vi "Load_Analogue_Data_2_Time_traces.vi"(0 "Sampling Rate (Hz)":dbl[](array[numeric]), 1 "Mode":T1, 2 "Index":i32[](array[numeric]), 3 "Voltage Array":dbl[][](array[numeric]), 4 "Time Trace":T2[](array[typedef]), 5 "Metadata Names":string[][](array[string]), 6 "Metadata Values":string[][](array[string])) -> ()   [LabVIEW 2021]
uses:
  Controls/Time_Trace_Cluster.ctl
  Sub_vis/Upload Data.ctl
  Globals/Meas_global.vi
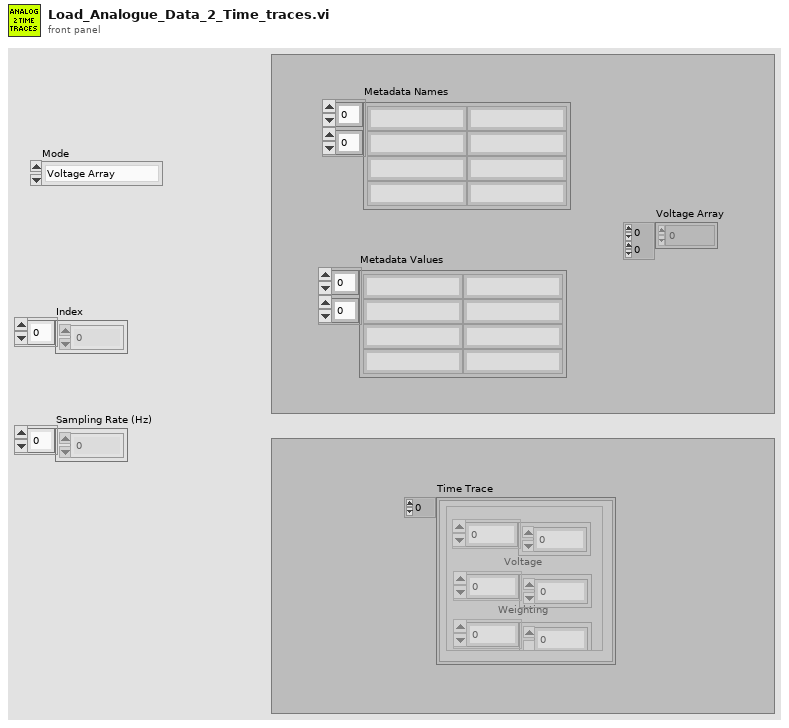
[diagram p1: front panel]
types:
  T1 = typedef "Upload Data.ctl" = enum16{"Voltage Array", "Time Trace Cluster"}
  T2 = typedef "Time_Trace_Cluster.ctl" = cluster{"Weighting":dbl[], "Voltage":dbl[], "Eng Values":dbl[]}
  T3 = typedef "Analysis_info_cluster.ctl" = cluster{"Colour":u32, "Inst type":T4, "Inst name":string, "Symbol":string, "Code name":string, "Extra Info":string, "Inst Array":T5, "Extra Titles":string[], "Extra Values":string[], "U":dbl, "u^2":dbl, "u^3":dbl, "u^4":dbl, "Skew_u":dbl, "Kurt_u":dbl, "Sd Error in Mean":dbl, "% u'/U":dbl, "X":dbl, "Y":dbl, "Z":dbl, "Timescale integral Estimate":dbl, "Sd Error in Variance":dbl, "Calib File":path, "Calib Constants":dbl[], "Output Position":bool, "Stats":enum16{"None", "Basic", "Full"}, "Av Sampling Rate":dbl, "Av No of Samples":dbl, "Total Meas Time (s)":dbl, "ADAM Ch Name":string, "Max value":dbl, "Min value":dbl, "Req Sample Rate Hz":dbl, "Sync Delay Time (s)":dbl, "Ch No":i16, "Device":string, "Use Latest Calib":bool, "Port":string, "Metadata Ch Names":string[], "Metadata Ch Values":string[], "Label":string}
  T4 = typedef "Inst_type.ctl" = enum16{"Raw voltage", "Raw with zero offsetting", "Propeller anemometer", "Pressure Transducer", "Pitot-static tube", "Hot wire", "Cross wire 1", "Cross wire 2", "Generic Linear", "Generic Polynomial", "Generic BackPoly", "Fast FID", "Thermocouple", "Cold wire", "Pulsed Wire", "LDA Vel", "LDA Tran time", "LDA Arr time", "Microphone"}
  T5 = typedef "Instrument_Array.ctl" = enum16{"PWA", "LDA", "Analogue"}
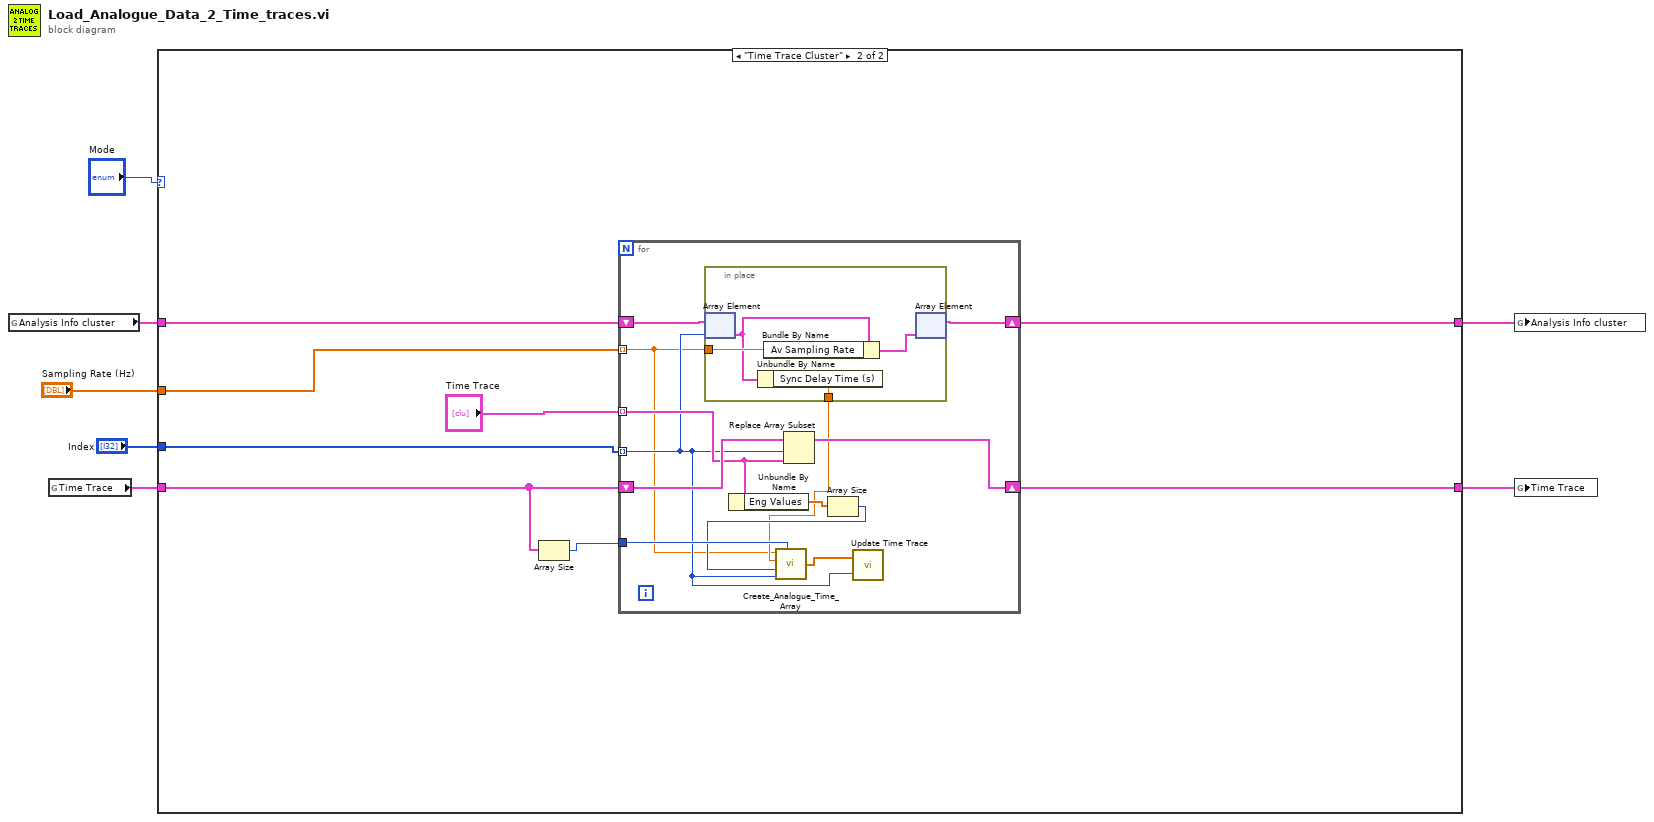
[diagram p0: block diagram]
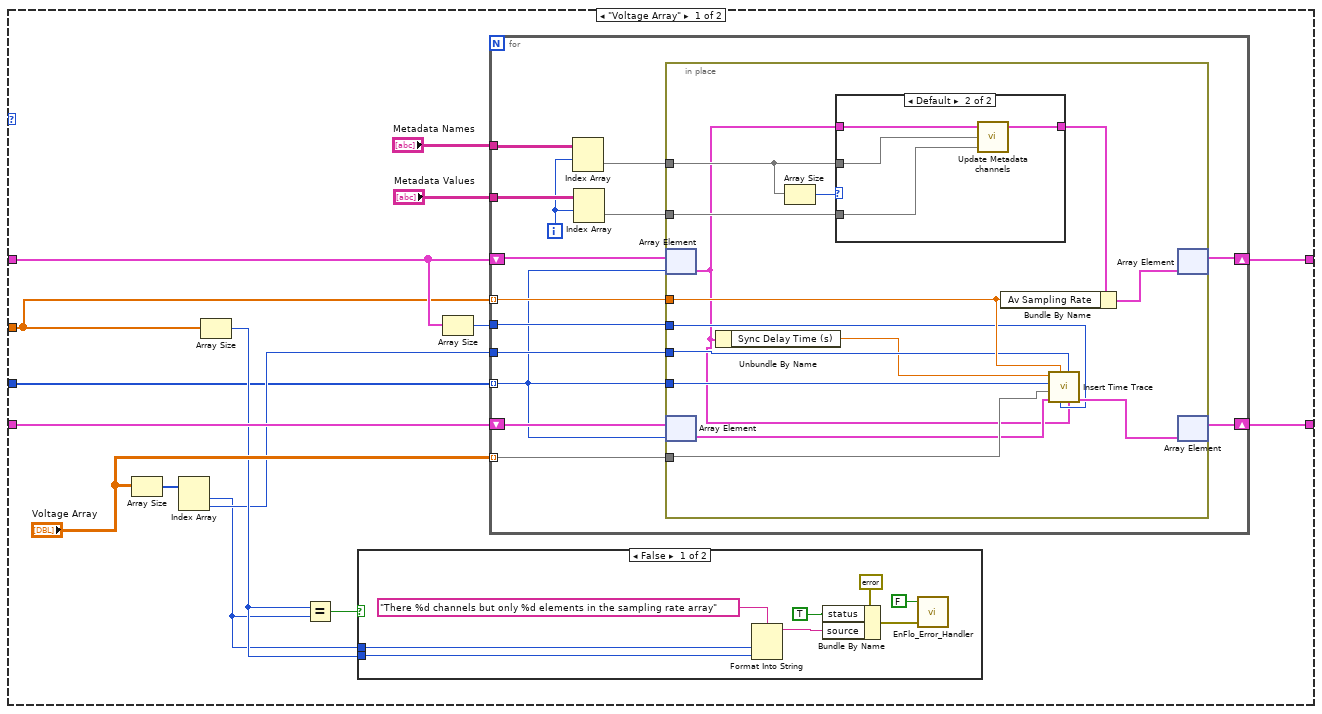
[diagram p2: hidden frame]
diagram:
  n1 = global read "Meas_global.vi" "Analysis Info cluster"() -> (w4:T3[])
  n2 = global read "Meas_global.vi" "Time Trace"() -> (w6:T2[])
  n3 = case shown="\"Time Trace Cluster\"" "Mode" {
    tunnel: [w22 w69] -> w7
    tunnel: w6 -> [w21 w65]
    tunnel: [w14 w70] -> w5
    tunnel: w4 -> [w13 w71]
    tunnel: "Sampling Rate (Hz)" -> [w9 w68]
    tunnel: "Index" -> [w8 w66]
    frame "Voltage Array" {
      n4 = Array Size(array="Voltage Array") -> (size(s)=w19:i32[])
      n5 = Index Array(array=w19) -> (element #1=w15:i32, element #2=w16:i32)  [unwired: 2 in]
      n6 = Array Size(array=w9) -> (size(s)=w17:i32)
      n7 = Equal?(x=w17, y=w15) -> (x = y?=w18:bool)
      n8 = case shown="False" w18 {
        tunnel: w15 -> [w27 _]
        tunnel: w17 -> [w26 _]
        frame False {
          n9 = Format Into String(format string="There %d channels but only %d elements in the sampling rate array", w27, w26) -> (resulting string=w24:string)  [unwired: 2 in, 1 out]
          n10 = Bundle By Name(cluster=errorcluster {"status"=FALSE, "code"=0, "source"=""} ("error in (no error)"), "status"=TRUE, "source"=w24) -> (w23:errorcluster)
          n11 = call "EnFlo_Error_Handler.vi"("error in (no error)"=w23, "Dialog Box (F)"=FALSE ("Dialog Box (T)")) -> ()  [unwired: 2 in, 2 out]
        }
        frame True {
        }
      }
      n12 = Array Size(array=w13) -> (size(s)=w12:i32)
      n13 = for {
        shift-right: [w42] -> w22
        shift-left: w21 -> [w44]
        tunnel: w8 -> [w36] mode=indexing
        tunnel: "Voltage Array" -> [w43] mode=indexing
        tunnel: w9 -> [w41] mode=indexing
        tunnel: w16 -> [w40]
        tunnel: w12 -> [w39]
        shift-right: [w37] -> w14
        shift-left: w13 -> [w38]
        tunnel: "Metadata Names" -> [w32]
        tunnel: "Metadata Values" -> [w35]
        i -> [w33]
        n14 = Index Array(array=w32, index (row)=w33) -> (element=w31:string[])  [unwired: 1 in]
        n15 = Index Array(array=w35, index (row)=w33) -> (element=w34:string[])  [unwired: 1 in]
        n16 = in-place {
          in-place-border: w43 -> [w53]
          in-place-border: w41 -> [w50]
          in-place-border: w40 -> [w49]
          in-place-border: w39 -> [w46]
          in-place-border: w36 -> [w47]
          in-place-border: w31 -> [w55]
          in-place-border: w34 -> [w57]
          n17 = in-place-array #1(w38, w36) -> (w45:T3)
          n18 = in-place-array #2(w44, w36) -> (w52:T2)
          n19 = Unbundle By Name(w45) -> ("Sync Delay Time (s)"=w48:dbl)
          n20 = Array Size(array=w55) -> (size(s)=w54:i32)
          n21 = case shown="Default" w54 {
            tunnel: w45 -> [w59 w63]
            tunnel: w57 -> [_ w60]
            tunnel: [w59 w62] -> w56
            tunnel: w55 -> [_ w61]
            frame 0 {
            }
            frame Default {
              n22 = call "Update Metadata channels.vi"("Metadata Values"=w60, "Metadata Names"=w61, "Analysis info Cluster in"=w63) -> ("Analysis info Cluster out"=w62:T3)
            }
          }
          n23 = Bundle By Name(cluster=w56, "Av Sampling Rate"=w50) -> (w58:T3)
          n24 = call "Insert Time Trace.vi"("Anlaysis Info Cluster"=w45, "No of Samples"=w49, "Total No of Chs"=w46, "Sampling Rate (Hz)"=w50, "Time Trace In"=w52, "Input Array"=w53, "Index"=w47, "Sync Delay (s)"=w48) -> ("Time Trace Out"=w51:T2)  [unwired: 3 in]
          n25 = in-place-array #1(w58) -> (w37:T3[])  [unwired: 1 out]
          n26 = in-place-array #2(w51) -> (w42:T2[])  [unwired: 1 out]
        }
      }
    }
    frame "Time Trace Cluster" {
      n27 = Array Size(array=w65) -> (size(s)=w64:i32)
      n28 = for {
        shift-right: [w82] -> w69
        shift-left: w65 -> [w83]
        tunnel: "Time Trace" -> [w77] mode=indexing
        tunnel: w66 -> [w74] mode=indexing
        shift-right: [w80] -> w70
        shift-left: w71 -> [w81]
        tunnel: w68 -> [w72] mode=indexing
        tunnel: w64 -> [w78]
        n29 = in-place {
          in-place-border: w72 -> [w86]
          in-place-border: [w84] -> w73
          n30 = in-place-array #3(w81, w74) -> (w85:T3)
          n31 = Unbundle By Name(w85) -> ("Sync Delay Time (s)"=w84:dbl)
          n32 = Bundle By Name(cluster=w85, "Av Sampling Rate"=w86) -> (w87:T3)
          n33 = in-place-array #3(w87) -> (w80:T3[])  [unwired: 1 out]
        }
        n34 = Unbundle By Name(w77) -> ("Eng Values"=w76:dbl[])
        n35 = Replace Array Subset(array=w83, new element=w77, index=w74) -> (w82:T2[])
        n36 = Array Size(array=w76) -> (size(s)=w75:i32)
        n37 = call "Create_Analogue_Time_Array.vi"("Sampling Rate (Hz)"=w72, "Sync Delay (s)"=w73, "No of Samples"=w75, "Index"=w74, "Total No of Chs"=w78) -> ("Times"=w79:dbl[])
        n38 = call "Update Time Trace.vi"("Channel Index"=w74, "Time (s)"=w79) -> ()  [unwired: 1 in]
      }
    }
  }
  n39 = global write "Meas_global.vi" "Analysis Info cluster"(w5) -> ()
  n40 = global write "Meas_global.vi" "Time Trace"(w7) -> ()
